vi "XIPIN_Local_Memory_Bus_(LMB)_1.0_3_0.vi"   [LabVIEW 2017]
doc: "The LMB is a fast, local bus for connecting MicroBlaze I and D ports to peripherals and BRAM\n------------------------------------\n<b>Need License</b> : No"
uses:
  <vilib>/rvi/XilinxIP/XIPIN_XNode/niFpgaXIPIN.xnode
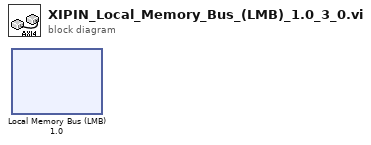
[diagram p0: block diagram]
diagram:
  n1 = xnode ("Local Memory Bus (LMB) 1.0")() -> ()
